vi "Close.vi"(8 "error in (no error)":errorcluster, 11 "NI DA in":refnum<class "NI Digital to Analog.lvclass">) -> (0 "error out":errorcluster, 3 "NI DA out":refnum<class "NI Digital to Analog.lvclass">)   [LabVIEW 2024, in "NI Digital to Analog.lvclass"]
doc: "Bus.lvclass:Close.vi\n\nThis is the template for the Close VI for the bus class.\n\nInstrument Communication Module Version 1.0\nJuly, 2017 Original Code Consulting David Thomson\n www.originalcode.com"
uses:
  NI Digital to Analog.lvclass
  NI Digital to Analog.lvclass/NI Digital to Analog.ctl
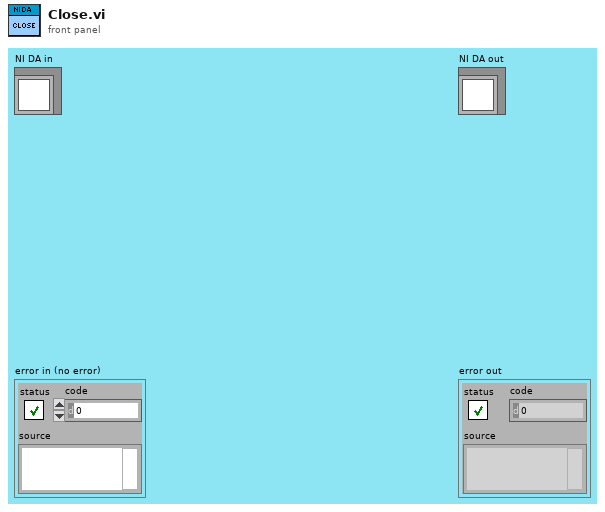
[diagram p1: front panel]
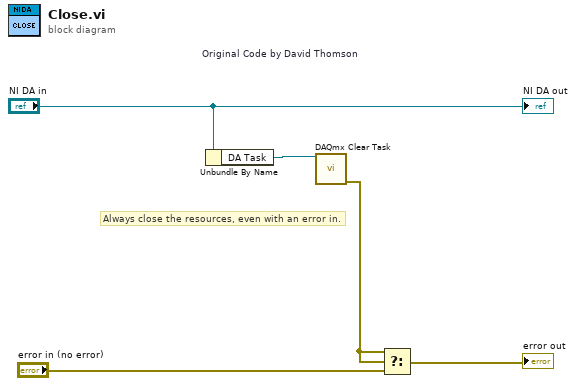
[diagram p0: block diagram]
diagram:
  # "Always close the resources, even with an error in."
  n1 = Unbundle By Name "Original Code by David Thomson"("NI DA in") -> ("DA Task"=w4:refnum<k21>)
  n2 = call "DAQmx Clear Task.vi"("task in"=w4) -> ("error out"=w3:errorcluster)  [unwired: 14 in]
  n3 = Select(t=w3, s=w3, f="error in (no error)") -> (s? t:f=→"error out":errorcluster)
  "NI DA out" <- "NI DA in"
